vi "as_genStimList.vi"(7 "Stimulus List Start Num":i32 caption="Stimulus List Numbering Start", 10 "Stimulus Parameters":dbl[][](array[numeric]), 11 "Repetitions":i32 caption="# of Random Repetitions for Each Stimulus" min=2) -> (2 "Stimulus List":dbl[][](array[numeric]))   [LabVIEW 2009]
panel:
  # "Stim#, Stim Type, Duration, Amplitude, Param 1, Param 2, Param 3, Param 4"
  # "Stim Type, Duration, Amplitude, Param 1, Param 2, Param 3, Param 4"
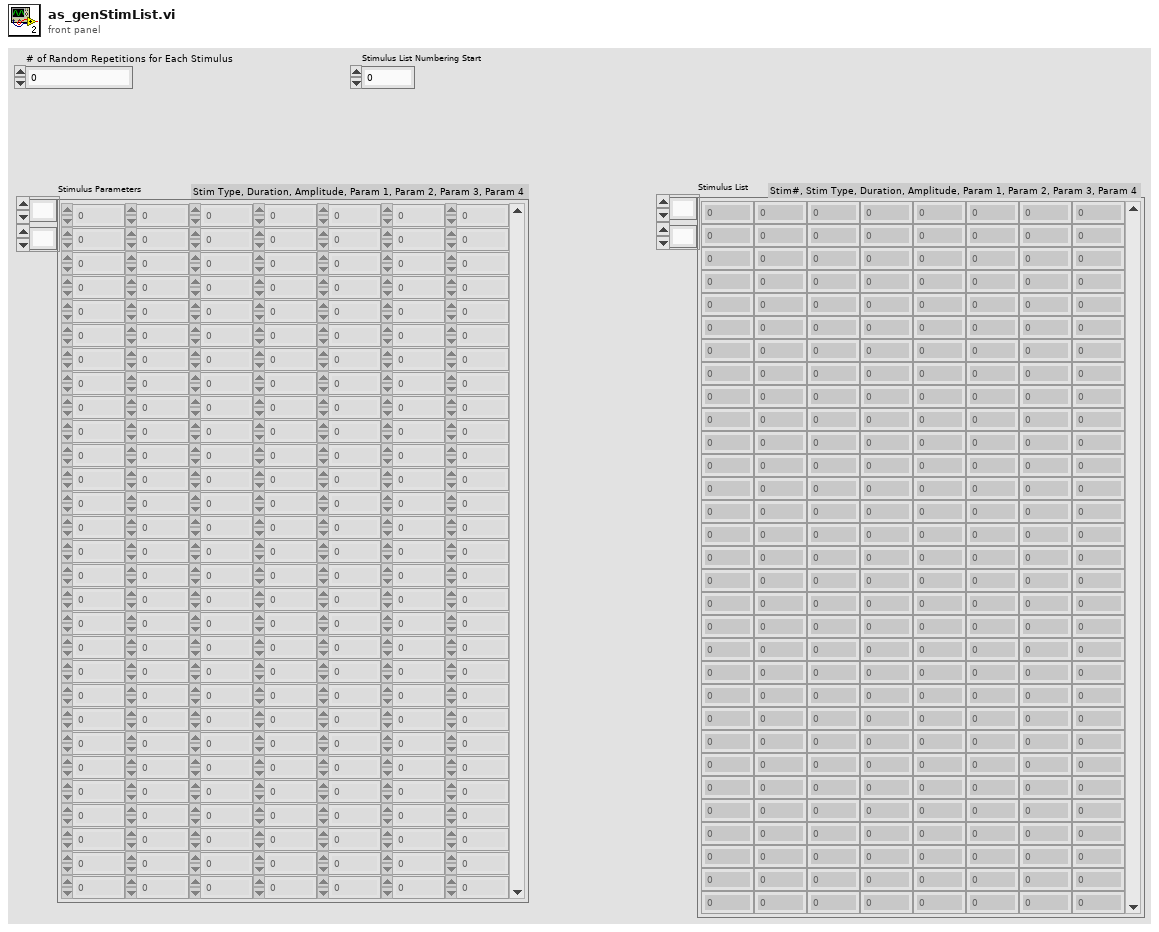
[diagram p1: front panel]
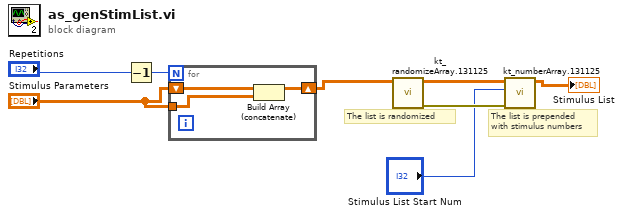
[diagram p0: block diagram]
diagram:
  # "The list is prepended\nwith stimulus numbers"
  # "The list is randomized"
  n1 = Decrement(x="Repetitions") -> (x-1=w8:i32)
  n2 = for {
    N: w8 -> [_]
    shift-right: [w11] -> w7
    shift-left: "Stimulus Parameters" -> [w10]
    tunnel: "Stimulus Parameters" -> [w9]
    n3 = Build Array (concatenate)(w10, w9) -> (w11:dbl[][])
  }
  n4 = call "kt_randomizeArray.131125.vi"("Array In"=w7) -> ("error out"=w5:errorcluster, "Array Out"=w6:dbl[][])  [unwired: 9 in]
  n5 = call "kt_numberArray.131125.vi"("error in (no error)"=w5, "Stimulus List Start Num"="Stimulus List Start Num", "Array In"=w6) -> ("Array Out"=→"Stimulus List":dbl[][])  [unwired: 7 in, 1 out]
